vi "Get Bundle Definition Tree.vi"(8 "error in (no error)":errorcluster, 11 "Bundle Builder in":refnum<class "Bundle Builder.lvclass">) -> (0 "error out":errorcluster, 1 "Tree Selection Types":string[](array[combo]), 2 "Tree Selections":string[](array[string]), 3 "Bundle Builder out":refnum<class "Bundle Builder.lvclass">)   [LabVIEW 2020, in "Bundle Builder.lvclass"]
uses:
  Bundle Builder.lvclass
  Bundle Builder.lvclass/Bundle Builder.ctl
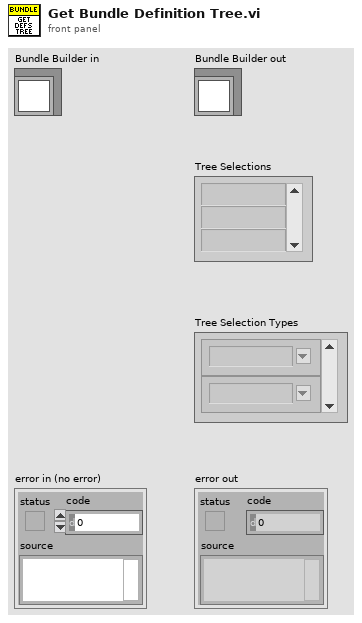
[diagram p1: front panel]
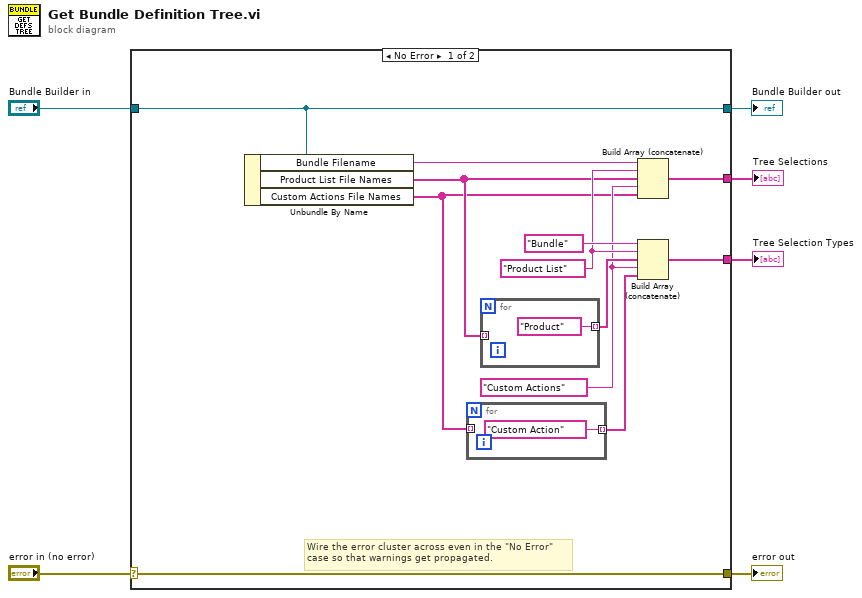
[diagram p0: block diagram]
diagram:
  n1 = case shown="No Error" "error in (no error)" {
    selector: "error in (no error)" -> [w18 w22]
    tunnel: [w18 w22] -> w5
    tunnel: [w17 w21] -> w3
    tunnel: "Bundle Builder in" -> [w17 w21]
    tunnel: [w8 _] -> w1
    tunnel: [w7 _] -> w2
    frame No Error {
      w10 = "Custom Actions" ("Selection Type")
      w12 = "Product List" ("Selection Type")
      # "Wire the error cluster across even in the \"No Error\"\ncase so that warnings get propagated."
      n2 = Unbundle By Name(w17) -> ("Bundle Filename"=w13:string, "Product List File Names"=w11:string[], "Custom Actions File Names"=w9:string[])
      n3 = for {
        tunnel: w9 -> [_] mode=indexing
        tunnel: ["Custom Action" ("Selection Type")] -> w14 mode=indexing
      }
      n4 = for {
        tunnel: w11 -> [_] mode=indexing
        tunnel: ["Product" ("Selection Type")] -> w15 mode=indexing
      }
      n5 = Build Array (concatenate)(w13, w12, w11, w10, w9) -> (w8:string[])
      n6 = Build Array (concatenate)("Bundle" ("Selection Type"), w12, w15, w10, w14) -> (w7:string[])
    }
    frame Error {
    }
  }
  "error out" <- w5
  "Bundle Builder out" <- w3
  "Tree Selection Types" <- w2
  "Tree Selections" <- w1
